vi "H2_v02.vi"(2 "Debug Mode":bool, 3 "Elapsed Time (s)":dbl, 4 "State":enum16{"Edit", "Start", "Run", "End", "Idle"}(ring), 5 "Argument List In":string[](array[string])) -> (0 "Status Out":string, 1 "Argument List Out":string[](array[string]))   [LabVIEW 2011]
panel:
  in  "AsH3 Run":bool
  in  "AsH3 Flow (0-10 sccm)":dbl format="%.2f"
  in  "P Flow (0-100 sccm)":dbl format="%.2f"
  in  "PH3 Run":bool
  in  "In Flow (0-100 sscm)":dbl format="%.2f"
  in  "In run":bool
  in  "Dilution factor":dbl min=0.0 max=10.0 format="%.2f"
  in  "Ga Run":bool
  in  "Ga Flow (0-10 sscm)":dbl format="%.2f"
  in  "Al Run":bool
  in  "Al Flow (0-100 sscm)":dbl format="%.2f"
  out "Al?":bool
  out "In?":bool
  out "Ga?":bool
  out "AsH3?":bool
  out "PH3?":bool
  in  "Cancel":bool
  in  "OK":bool
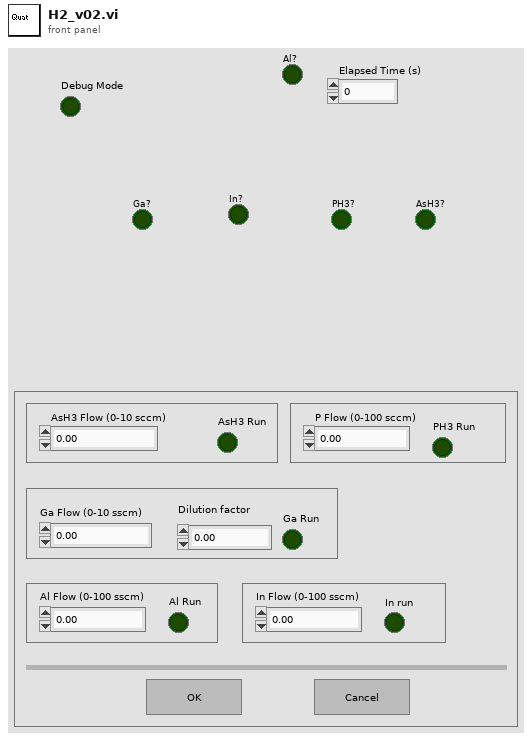
[diagram p1: front panel]
types:
  T1 = enum16{"Discrete", "Continuous", "Instantaneous"}
  T2 = enum32{"Invalid", "Default", "Floating", "Floating/Auto-Hide", "Modal"}
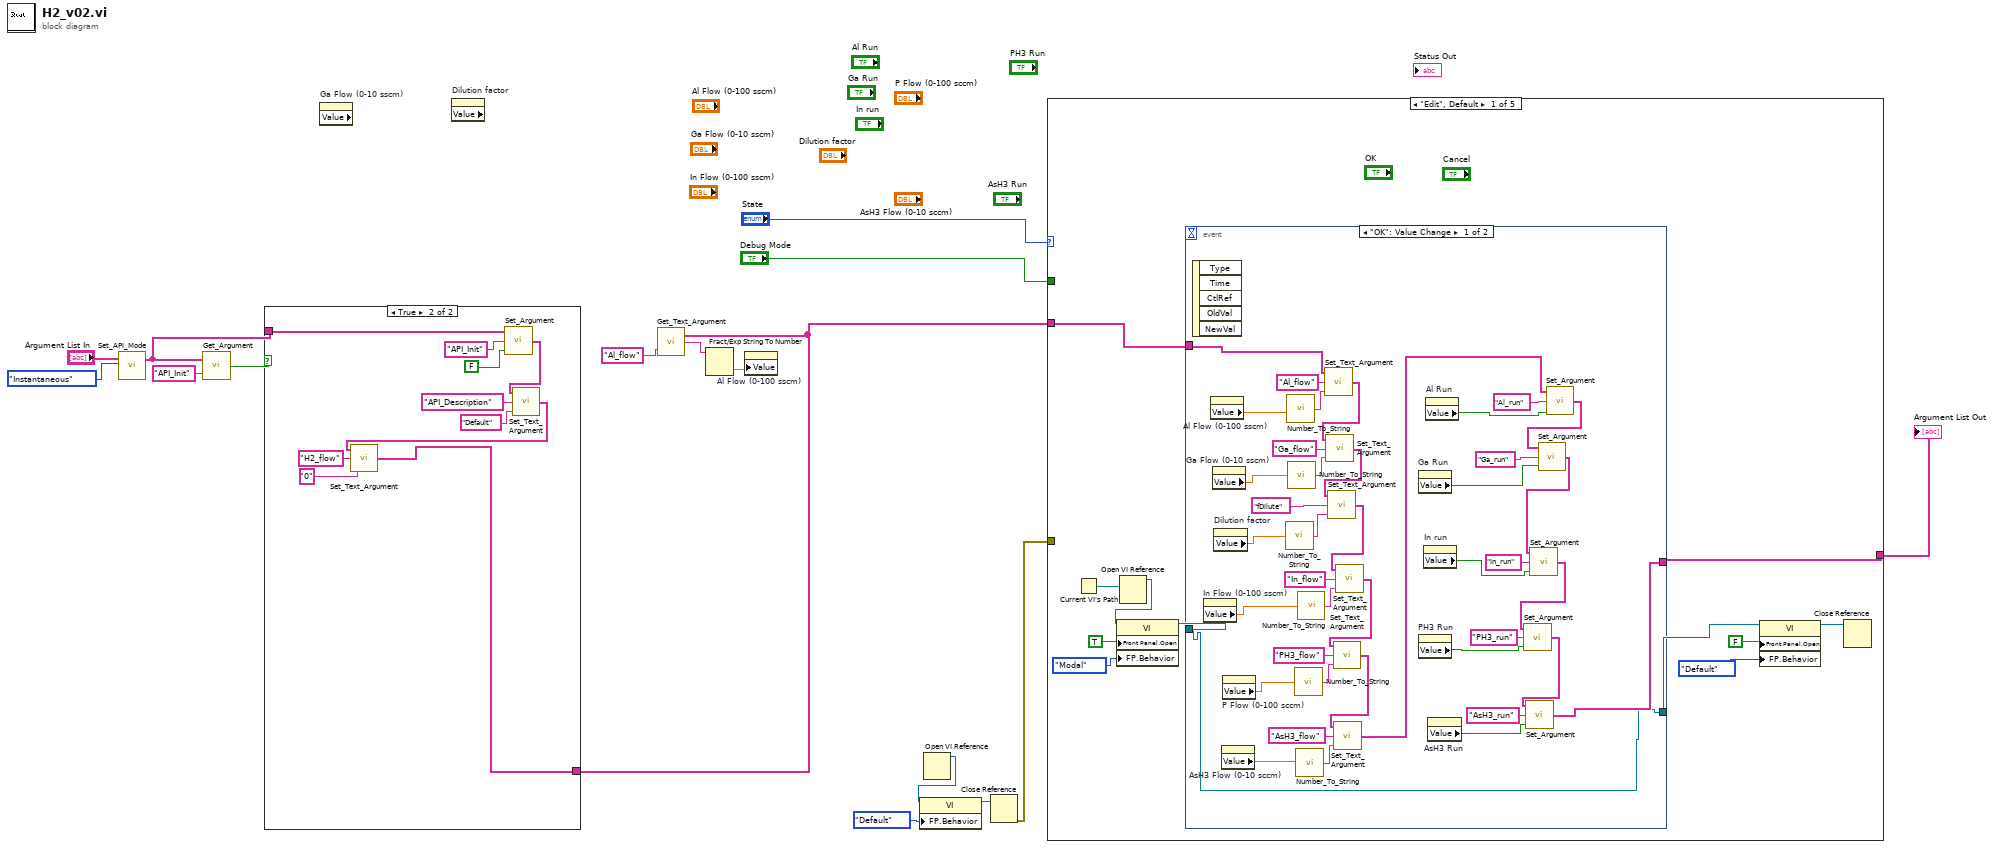
[diagram p0: block diagram]
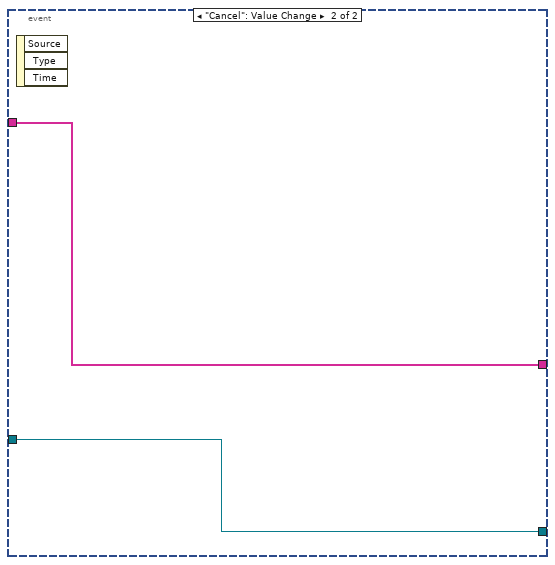
[diagram p3: hidden frame]
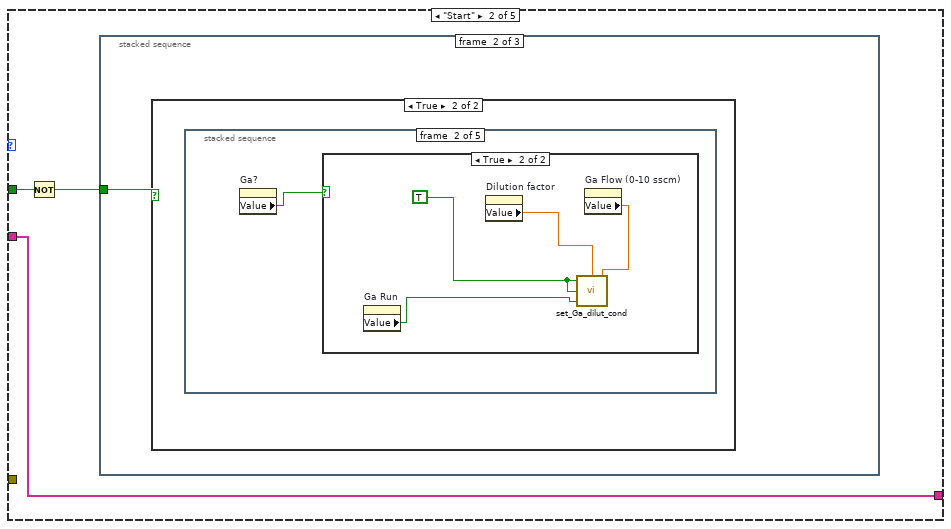
[diagram p4: hidden frame]
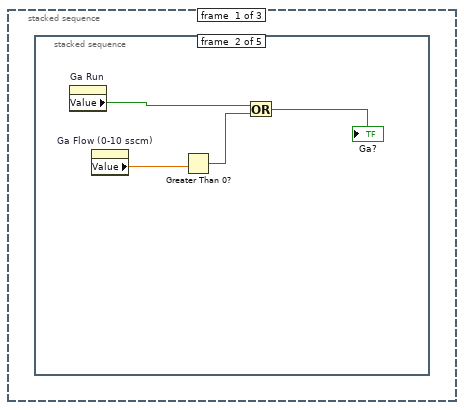
[diagram p5: hidden frame]
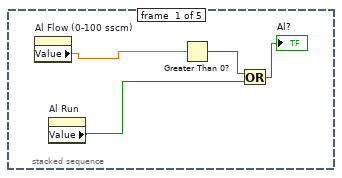
[diagram p6: hidden frame]
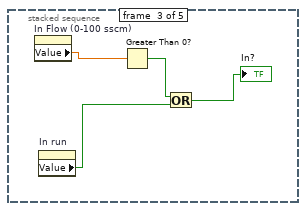
[diagram p7: hidden frame]
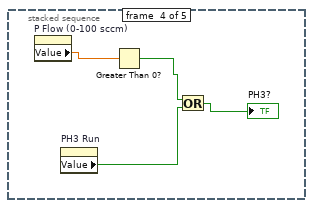
[diagram p8: hidden frame]
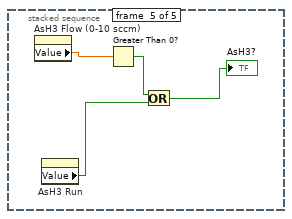
[diagram p9: hidden frame]
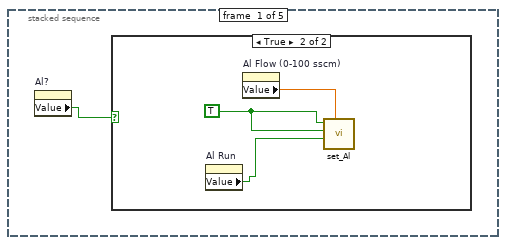
[diagram p11: hidden frame]
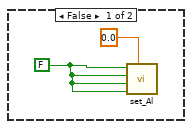
[diagram p12: hidden frame]
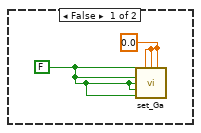
[diagram p13: hidden frame]
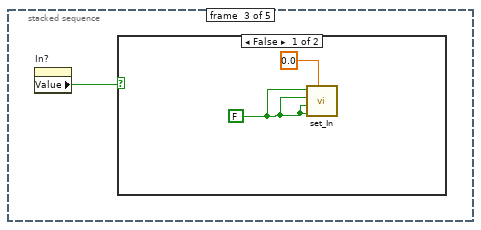
[diagram p14: hidden frame]
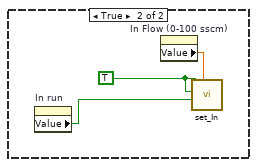
[diagram p15: hidden frame]
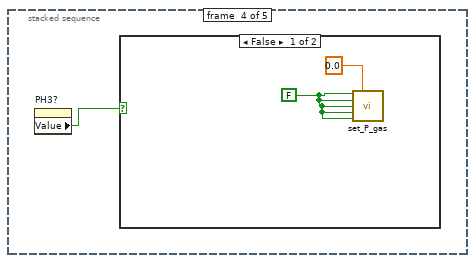
[diagram p16: hidden frame]
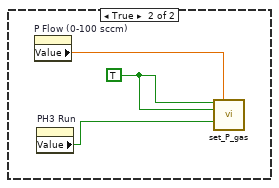
[diagram p17: hidden frame]
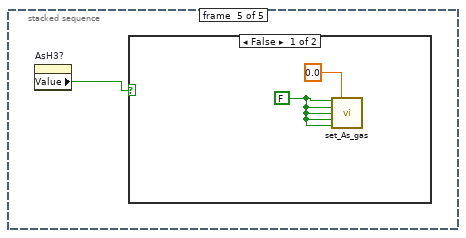
[diagram p18: hidden frame]
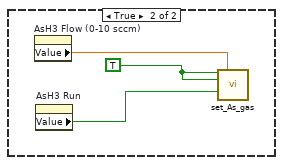
[diagram p19: hidden frame]
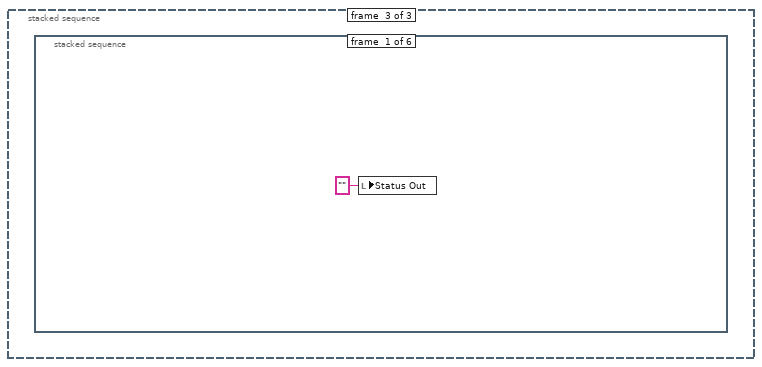
[diagram p20: hidden frame]
diagram:
  n1 = call "Set_API_Mode.vi"("API Mode"=T1."Instantaneous", "Argument List In"="Argument List In") -> ("Argument List Out"=w5:string[])  [unwired: 3 in]
  n2 = call "Get_Argument.vi"("Argument"="API_Init", "Argument List"=w5) -> ("Enabled"=w6:bool)
  n3 = case shown="True" w6 {
    tunnel: w5 -> [w18 w28]
    tunnel: [w18 w19] -> w1
    frame False {
    }
    frame True {
      n4 = call "Set_Argument.vi"("Enable"=FALSE, "Argument"="API_Init", "Argument List In"=w28) -> ("Argument List Out"=w25:string[])
      n5 = call "Set_Text_Argument.vi"("Text"="Default", "Argument"="API_Description", "Argument List In"=w25) -> ("Argument List Out"=w20:string[])
      n6 = call "Set_Text_Argument.vi"("Text"="0", "Argument"="H2_flow", "Argument List In"=w20) -> ("Argument List Out"=w19:string[])
    }
  }
  n7 = property on="Ga Flow (0-10 sscm)" class="DigNum (strict)" props=["Value"]() -> ()  [unwired: 2 in, 3 out]
  n8 = property on="Dilution factor" class="DigNum (strict)" props=["Value"]() -> ()  [unwired: 2 in, 3 out]
  n9 = call "Get_Text_Argument.vi"("Argument"="Al_flow", "Argument List"=w1) -> ("Text"=w3:string)
  n10 = Fract/Exp String To Number(string=w3) -> (number=w2:dbl)  [unwired: 4 out]
  n11 = property on="Al Flow (0-100 sscm)" class="DigNum (strict)"("Value"=w2) -> ()  [unwired: 2 in, 2 out]
  n12 = Open VI Reference() -> (vi path=w14:path, vi reference=w13:refnum<vi>)  [unwired: 1 in, 5 out]
  n13 = property class="VI"(reference=w13, "FP.Behavior"=T2."Default" ("Front Panel Window:Behavior")) -> (reference out=w11:refnum<vi>)  [unwired: 1 in, 1 out]
  n14 = Close Reference(reference=w11) -> (error out=w10:errorcluster)  [unwired: 1 in]
  n15 = case shown="\"Edit\", Default" "State" {
    tunnel: [w39 w85 w208 w209 w210] -> w16
    tunnel: w1 -> [w38 w85 w208 w209 w210]
    tunnel: "Debug Mode" -> [_ w84 _ _ _]
    tunnel: w10 -> [_ _ _ _ _]
    frame "Edit", Default {
      n16 = Current VI's Path() -> (path=w33:path)
      n17 = Open VI Reference(vi path=w33) -> (vi reference=w32:refnum<vi>)  [unwired: 1 in, 5 out]
      n18 = property class="VI"(reference=w32, "Front Panel.Open"=TRUE ("Front Panel Window:Open"), "FP.Behavior"=T2."Modal" ("Front Panel Window:Behavior")) -> (reference out=w36:refnum<vi>)  [unwired: 1 in, 1 out]
      n19 = event shown="[0] \"OK\": Value Change" {
        selector: _ -> [_ _]
        dyn-events: _ -> [_ _]
        timeout: _ -> [_ _]
        tunnel: w38 -> [w63 w81]
        tunnel: [w68 w81] -> w39
        tunnel: [w55 w82] -> w35
        tunnel: w36 -> [w55 w82]
        event "OK": Value Change {
          n20 = event-data() -> ()  [unwired: 6 out]
          n21 = property on="In Flow (0-100 sscm)" class="DigNum (strict)"() -> ("Value"=w47:dbl)  [unwired: 2 in, 2 out]
          n22 = property on="Al Flow (0-100 sscm)" class="DigNum (strict)"() -> ("Value"=w50:dbl)  [unwired: 2 in, 2 out]
          n23 = property on="Ga Flow (0-10 sscm)" class="DigNum (strict)"() -> ("Value"=w49:dbl)  [unwired: 2 in, 2 out]
          n24 = property on="Dilution factor" class="DigNum (strict)"() -> ("Value"=w48:dbl)  [unwired: 2 in, 2 out]
          n25 = property on="AsH3 Flow (0-10 sccm)" class="DigNum (strict)"() -> ("Value"=w45:dbl)  [unwired: 2 in, 2 out]
          n26 = property on="P Flow (0-100 sccm)" class="DigNum (strict)"() -> ("Value"=w46:dbl)  [unwired: 2 in, 2 out]
          n27 = call "Number_To_String.vi"("Number"=w48) -> ("String"=w52:string)
          n28 = call "Number_To_String.vi"("Number"=w50) -> ("String"=w64:string)
          n29 = call "Number_To_String.vi"("Number"=w49) -> ("String"=w79:string)
          n30 = call "Number_To_String.vi"("Number"=w46) -> ("String"=w75:string)
          n31 = call "Number_To_String.vi"("Number"=w45) -> ("String"=w60:string)
          n32 = call "Number_To_String.vi"("Number"=w47) -> ("String"=w77:string)
          n33 = call "Set_Text_Argument.vi"("Text"=w64, "Argument"="Al_flow", "Argument List In"=w63) -> ("Argument List Out"=w62:string[])
          n34 = call "Set_Text_Argument.vi"("Text"=w79, "Argument"="Ga_flow", "Argument List In"=w62) -> ("Argument List Out"=w53:string[])
          n35 = call "Set_Text_Argument.vi"("Text"=w52, "Argument"="fDilute", "Argument List In"=w53) -> ("Argument List Out"=w54:string[])
          n36 = call "Set_Text_Argument.vi"("Text"=w77, "Argument"="In_flow", "Argument List In"=w54) -> ("Argument List Out"=w57:string[])
          n37 = call "Set_Text_Argument.vi"("Text"=w75, "Argument"="PH3_flow", "Argument List In"=w57) -> ("Argument List Out"=w58:string[])
          n38 = call "Set_Text_Argument.vi"("Text"=w60, "Argument"="AsH3_flow", "Argument List In"=w58) -> ("Argument List Out"=w59:string[])
          n39 = property on="Ga Run" class="Bool (strict)"() -> ("Value"=w41:bool)  [unwired: 2 in, 2 out]
          n40 = property on="PH3 Run" class="Bool (strict)"() -> ("Value"=w43:bool)  [unwired: 2 in, 2 out]
          n41 = property on="In run" class="Bool (strict)"() -> ("Value"=w42:bool)  [unwired: 2 in, 2 out]
          n42 = property on="Al Run" class="Bool (strict)"() -> ("Value"=w40:bool)  [unwired: 2 in, 2 out]
          n43 = property on="AsH3 Run" class="Bool (strict)"() -> ("Value"=w44:bool)  [unwired: 2 in, 2 out]
          n44 = call "Set_Argument.vi"("Enable"=w40, "Argument"="Al_run", "Argument List In"=w59) -> ("Argument List Out"=w56:string[])
          n45 = call "Set_Argument.vi"("Enable"=w41, "Argument"="Ga_run", "Argument List In"=w56) -> ("Argument List Out"=w71:string[])
          n46 = call "Set_Argument.vi"("Enable"=w42, "Argument"="In_run", "Argument List In"=w71) -> ("Argument List Out"=w66:string[])
          n47 = call "Set_Argument.vi"("Enable"=w43, "Argument"="PH3_run", "Argument List In"=w66) -> ("Argument List Out"=w67:string[])
          n48 = call "Set_Argument.vi"("Enable"=w44, "Argument"="AsH3_run", "Argument List In"=w67) -> ("Argument List Out"=w68:string[])
        }
        event "Cancel": Value Change {
          n49 = event-data() -> ()  [unwired: 4 out]
        }
      }
      n50 = property class="VI"(reference=w35, "Front Panel.Open"=FALSE ("Front Panel Window:Open"), "FP.Behavior"=T2."Default" ("Front Panel Window:Behavior")) -> (reference out=w29:refnum<vi>)  [unwired: 1 in, 1 out]
      n51 = Close Reference(reference=w29) -> ()  [unwired: 1 in, 1 out]
    }
    frame "Start" {
      n52 = Not(x=w84) -> (.not. x?=w83:bool)
      n53 = stacked-sequence {
        tunnel: w83 -> [_ w106 _]
        frame #0 {
          n54 = stacked-sequence {
            frame #0 {
              n55 = property on="Al Flow (0-100 sscm)" class="DigNum (strict)"() -> ("Value"=w87:dbl)  [unwired: 2 in, 2 out]
              n56 = property on="Al Run" class="Bool (strict)"() -> ("Value"=w86:bool)  [unwired: 2 in, 2 out]
              n57 = Greater Than 0?(x=w87) -> (x > 0?=w89:bool)
              n58 = Or(x=w89, y=w86) -> (x .or. y?=→"Al?":bool)
            }
            frame #1 {
              n59 = property on="Ga Run" class="Bool (strict)"() -> ("Value"=w92:bool)  [unwired: 2 in, 2 out]
              n60 = property on="Ga Flow (0-10 sscm)" class="DigNum (strict)"() -> ("Value"=w90:dbl)  [unwired: 2 in, 2 out]
              n61 = Greater Than 0?(x=w90) -> (x > 0?=w91:bool)
              n62 = Or(x=w92, y=w91) -> (x .or. y?=→"Ga?":bool)
            }
            frame #2 {
              n63 = property on="In Flow (0-100 sscm)" class="DigNum (strict)"() -> ("Value"=w97:dbl)  [unwired: 2 in, 2 out]
              n64 = property on="In run" class="Bool (strict)"() -> ("Value"=w95:bool)  [unwired: 2 in, 2 out]
              n65 = Greater Than 0?(x=w97) -> (x > 0?=w96:bool)
              n66 = Or(x=w96, y=w95) -> (x .or. y?=→"In?":bool)
            }
            frame #3 {
              n67 = property on="P Flow (0-100 sccm)" class="DigNum (strict)"() -> ("Value"=w101:dbl)  [unwired: 2 in, 2 out]
              n68 = property on="PH3 Run" class="Bool (strict)"() -> ("Value"=w99:bool)  [unwired: 2 in, 2 out]
              n69 = Greater Than 0?(x=w101) -> (x > 0?=w100:bool)
              n70 = Or(x=w100, y=w99) -> (x .or. y?=→"PH3?":bool)
            }
            frame #4 {
              n71 = property on="AsH3 Flow (0-10 sccm)" class="DigNum (strict)"() -> ("Value"=w105:dbl)  [unwired: 2 in, 2 out]
              n72 = property on="AsH3 Run" class="Bool (strict)"() -> ("Value"=w103:bool)  [unwired: 2 in, 2 out]
              n73 = Greater Than 0?(x=w105) -> (x > 0?=w104:bool)
              n74 = Or(x=w104, y=w103) -> (x .or. y?=→"AsH3?":bool)
            }
          }
        }
        frame #1 {
          n75 = case shown="True" w106 {
            frame False {
            }
            frame True {
              n76 = stacked-sequence {
                frame #0 {
                  n77 = property on="Al?" class="Bool (strict)"() -> ("Value"=w107:bool)  [unwired: 2 in, 2 out]
                  n78 = case shown="True" w107 {
                    frame False {
                      w108 = FALSE ("Al Active")
                      n79 = call "set_Al.vi"("Aluminum Flow"=0.0, "Al Remote"=w108, "Al Run"=w108, "Al Bubbler"=w108, "Al Active"=w108) -> ()  [unwired: 5 out]
                    }
                    frame True {
                      w112 = TRUE ("Al Active")
                      n80 = property on="Al Run" class="Bool (strict)"() -> ("Value"=w110:bool)  [unwired: 2 in, 2 out]
                      n81 = property on="Al Flow (0-100 sscm)" class="DigNum (strict)"() -> ("Value"=w111:dbl)  [unwired: 2 in, 2 out]
                      n82 = call "set_Al.vi"("Aluminum Flow"=w111, "Al Run"=w110, "Al Bubbler"=w112, "Al Active"=w112) -> ()  [unwired: 1 in, 5 out]
                    }
                  }
                }
                frame #1 {
                  n83 = property on="Ga?" class="Bool (strict)"() -> ("Value"=w113:bool)  [unwired: 2 in, 2 out]
                  n84 = case shown="True" w113 {
                    frame False {
                      w115 = FALSE ("Ga Active")
                      w114 = 0.0 ("Ga Flow 1")
                      n85 = call "set_Ga.vi"("Ga Active"=w115, "Ga Flow 3"=w114, "Ga Flow 2"=w114, "Ga Flow 1"=w114, "Ga Bubbler"=w115, "Ga H2 Dilute"=w115, "Ga Run"=w115, "Ga Remote"=w115) -> ()  [unwired: 8 out]
                    }
                    frame True {
                      w118 = TRUE ("Ga Active")
                      n86 = property on="Ga Run" class="Bool (strict)"() -> ("Value"=w119:bool)  [unwired: 2 in, 2 out]
                      n87 = property on="Dilution factor" class="DigNum (strict)"() -> ("Value"=w117:dbl)  [unwired: 2 in, 2 out]
                      n88 = property on="Ga Flow (0-10 sscm)" class="DigNum (strict)"() -> ("Value"=w116:dbl)  [unwired: 2 in, 2 out]
                      n89 = call "set_Ga_dilut_cond.vi"("Ga flow (0-10 sccm)"=w116, "fDilution"=w117, "Run"=w119, "Bubbler In"=w118, "Active"=w118) -> ()
                    }
                  }
                }
                frame #2 {
                  n90 = property on="In?" class="Bool (strict)"() -> ("Value"=w120:bool)  [unwired: 2 in, 2 out]
                  n91 = case shown="False" w120 {
                    frame False {
                      w122 = FALSE ("In Remote")
                      n92 = call "set_In.vi"("Indium Flow"=0.0, "In Remote"=w122, "In Run"=w122, "In Bubbler"=w122, "In Active"=w122) -> ()  [unwired: 5 out]
                    }
                    frame True {
                      w125 = TRUE ("In Run")
                      n93 = property on="In run" class="Bool (strict)"() -> ("Value"=w123:bool)  [unwired: 2 in, 2 out]
                      n94 = property on="In Flow (0-100 sscm)" class="DigNum (strict)"() -> ("Value"=w124:dbl)  [unwired: 2 in, 2 out]
                      n95 = call "set_In.vi"("Indium Flow"=w124, "In Run"=w123, "In Bubbler"=w125, "In Active"=w125) -> ()  [unwired: 1 in, 5 out]
                    }
                  }
                }
                frame #3 {
                  n96 = property on="PH3?" class="Bool (strict)"() -> ("Value"=w126:bool)  [unwired: 2 in, 2 out]
                  n97 = case shown="False" w126 {
                    frame False {
                      w127 = FALSE ("P_Gas Active")
                      n98 = call "set_P_gas.vi"("P_Gas Active"=w127, "P_Gas Flow"=0.0, "P_Gas In"=w127, "P_Gas H2 In"=w127, "P_Gas Run"=w127, "P_Gas Remote"=w127) -> ()  [unwired: 10 out]
                    }
                    frame True {
                      w131 = TRUE ("P_Gas Active")
                      n99 = property on="P Flow (0-100 sccm)" class="DigNum (strict)"() -> ("Value"=w130:dbl)  [unwired: 2 in, 2 out]
                      n100 = property on="PH3 Run" class="Bool (strict)"() -> ("Value"=w129:bool)  [unwired: 2 in, 2 out]
                      n101 = call "set_P_gas.vi"("P_Gas Active"=w131, "P_Gas Flow"=w130, "P_Gas In"=w131, "P_Gas Run"=w129) -> ()  [unwired: 2 in, 10 out]
                    }
                  }
                }
                frame #4 {
                  n102 = property on="AsH3?" class="Bool (strict)"() -> ("Value"=w132:bool)  [unwired: 2 in, 2 out]
                  n103 = case shown="False" w132 {
                    frame False {
                      w133 = FALSE ("As_Gas Active")
                      n104 = call "set_As_gas.vi"("As_Gas Active"=w133, "As_Gas Flow"=0.0, "As_Gas In"=w133, "As_Gas H2"=w133, "As_Gas Run"=w133, "As_Gas Remote"=w133) -> ()  [unwired: 10 out]
                    }
                    frame True {
                      w137 = TRUE ("As_Gas Active")
                      n105 = property on="AsH3 Flow (0-10 sccm)" class="DigNum (strict)"() -> ("Value"=w135:dbl)  [unwired: 2 in, 2 out]
                      n106 = property on="AsH3 Run" class="Bool (strict)"() -> ("Value"=w136:bool)  [unwired: 2 in, 2 out]
                      n107 = call "set_As_gas.vi"("As_Gas Active"=w137, "As_Gas Flow"=w135, "As_Gas In"=w137, "As_Gas Run"=w136) -> ()  [unwired: 2 in, 10 out]
                    }
                  }
                }
              }
            }
          }
        }
        frame #2 {
          n108 = stacked-sequence {
            frame #0 {
              n109 = local write "Status Out"("" ("Status Out")) -> ()
            }
            frame #1 {
              n110 = property on="Al Flow (0-100 sscm)" class="DigNum (strict)"() -> ("Value"=w140:dbl)  [unwired: 2 in, 2 out]
              n111 = property on="Al Run" class="Bool (strict)"() -> ("Value"=w139:bool)  [unwired: 2 in, 2 out]
              n112 = Format Into String(format string="%4.1f", w140) -> (resulting string=w143:string)  [unwired: 2 in, 1 out]
              n113 = case shown="True" w139 {
                tunnel: ["" ", run"] -> w146
                frame False {
                }
                frame True {
                }
              }
              n114 = Concatenate Strings("Al(" ("string"), w143, "sccm" ("string"), w146, ")" ("string")) -> (w144:string)
              n115 = property on="Al?" class="Bool (strict)"() -> ("Value"=w141:bool)  [unwired: 2 in, 2 out]
              n116 = case shown="True" w141 {
                tunnel: w144 -> [_ w149]
                frame False {
                }
                frame True {
                  n117 = local write "Status Out"(w149) -> ()
                }
              }
            }
            frame #2 {
              n118 = property on="Ga Run" class="Bool (strict)"() -> ("Value"=w154:bool)  [unwired: 2 in, 2 out]
              n119 = property on="Ga Flow (0-10 sscm)" class="DigNum (strict)"() -> ("Value"=w155:dbl)  [unwired: 2 in, 2 out]
              n120 = Format Into String(format string="%4.1f", w155) -> (resulting string=w157:string)  [unwired: 2 in, 1 out]
              n121 = case shown="True" w154 {
                tunnel: ["" ", run"] -> w160
                frame False {
                }
                frame True {
                }
              }
              n122 = property on="Status Out" class="Str"() -> ("Value"=w152:string)  [unwired: 2 in, 2 out]
              n123 = Concatenate Strings(w152, "Ga(" ("string"), w157, "sccm" ("string"), w160, ")" ("string")) -> (w158:string)
              n124 = property on="Ga?" class="Bool (strict)"() -> ("Value"=w153:bool)  [unwired: 2 in, 2 out]
              n125 = case shown="True" w153 {
                tunnel: w158 -> [_ w163]
                frame False {
                }
                frame True {
                  n126 = local write "Status Out"(w163) -> ()
                }
              }
            }
            frame #3 {
              n127 = property on="In run" class="Bool (strict)"() -> ("Value"=w168:bool)  [unwired: 2 in, 2 out]
              n128 = property on="In Flow (0-100 sscm)" class="DigNum (strict)"() -> ("Value"=w169:dbl)  [unwired: 2 in, 2 out]
              n129 = Format Into String(format string="%4.1f", w169) -> (resulting string=w171:string)  [unwired: 2 in, 1 out]
              n130 = property on="Status Out" class="Str"() -> ("Value"=w166:string)  [unwired: 2 in, 2 out]
              n131 = case shown="False" w168 {
                tunnel: ["" ", run"] -> w174
                frame False {
                }
                frame True {
                }
              }
              n132 = Concatenate Strings(w166, "In(" ("string"), w171, "sccm" ("string"), w174, ")" ("string")) -> (w172:string)
              n133 = property on="In?" class="Bool (strict)"() -> ("Value"=w167:bool)  [unwired: 2 in, 2 out]
              n134 = case shown="True" w167 {
                tunnel: w172 -> [_ w177]
                frame False {
                }
                frame True {
                  n135 = local write "Status Out"(w177) -> ()
                }
              }
            }
            frame #4 {
              n136 = property on="PH3 Run" class="Bool (strict)"() -> ("Value"=w183:bool)  [unwired: 2 in, 2 out]
              n137 = property on="P Flow (0-100 sccm)" class="DigNum (strict)"() -> ("Value"=w184:dbl)  [unwired: 2 in, 2 out]
              n138 = Format Into String(format string="%4.1f", w184) -> (resulting string=w186:string)  [unwired: 2 in, 1 out]
              n139 = case shown="False" w183 {
                tunnel: ["" ", run"] -> w188
                frame False {
                }
                frame True {
                }
              }
              n140 = property on="Status Out" class="Str"() -> ("Value"=w181:string)  [unwired: 2 in, 2 out]
              n141 = Concatenate Strings(w181, "PH3(" ("string"), w186, "sccm" ("string"), w188, ")" ("string")) -> (w182:string)
              n142 = property on="PH3?" class="Bool (strict)"() -> ("Value"=w185:bool)  [unwired: 2 in, 2 out]
              n143 = case shown="True" w185 {
                tunnel: w182 -> [_ w191]
                frame False {
                }
                frame True {
                  n144 = local write "Status Out"(w191) -> ()
                }
              }
            }
            frame #5 {
              n145 = property on="AsH3 Run" class="Bool (strict)"() -> ("Value"=w197:bool)  [unwired: 2 in, 2 out]
              n146 = property on="AsH3 Flow (0-10 sccm)" class="DigNum (strict)"() -> ("Value"=w198:dbl)  [unwired: 2 in, 2 out]
              n147 = Format Into String(format string="%4.2f", w198) -> (resulting string=w199:string)  [unwired: 2 in, 1 out]
              n148 = case shown="True" w197 {
                tunnel: ["" ", run"] -> w202
                frame False {
                }
                frame True {
                }
              }
              n149 = property on="Status Out" class="Str"() -> ("Value"=w195:string)  [unwired: 2 in, 2 out]
              n150 = Concatenate Strings(w195, "AsH3(" ("string"), w199, "sccm" ("string"), w202, ")" ("string")) -> (w200:string)
              n151 = property on="AsH3?" class="Bool (strict)"() -> ("Value"=w196:bool)  [unwired: 2 in, 2 out]
              n152 = case shown="True" w196 {
                tunnel: w200 -> [_ w205]
                frame False {
                }
                frame True {
                  n153 = local write "Status Out"(w205) -> ()
                }
              }
            }
          }
        }
      }
    }
    frame "Run" {
    }
    frame "End" {
    }
    frame "Idle" {
    }
  }
  "Argument List Out" <- w16
